vi "Operate LEDs.vi"(8 "error in (no error)":errorcluster, 10 "LED Panel":T1, 11 "COM port in":refnum<visa-resource-name>) -> (0 "error out":errorcluster, 3 "COM port out":refnum<visa-resource-name>)   [LabVIEW 2020]
uses:
  Controls/LED panel ---typedef.ctl
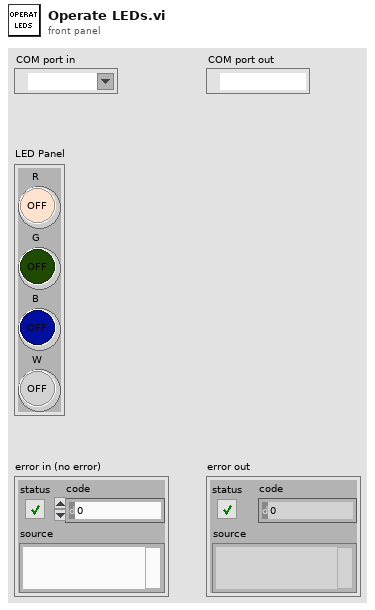
[diagram p1: front panel]
types:
  T1 = typedef "LED panel ---typedef.ctl" = cluster{"R":bool, "G":bool, "B":bool, "W":bool}
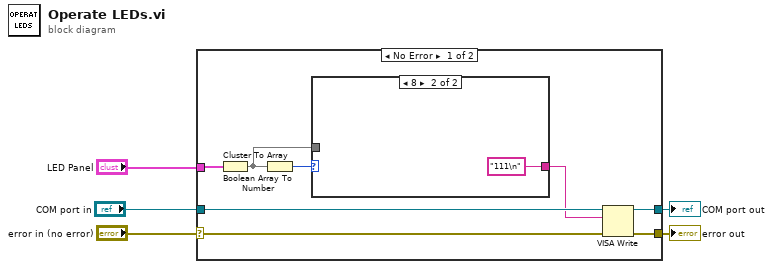
[diagram p0: block diagram]
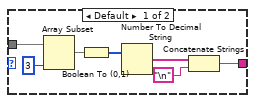
[diagram p2: hidden frame]
diagram:
  n1 = case shown="No Error" "error in (no error)" {
    selector: "error in (no error)" -> [w12 w23]
    tunnel: [w10 w23] -> w4
    tunnel: "LED Panel" -> [w13 _]
    tunnel: "COM port in" -> [w9 w22]
    tunnel: [w8 w22] -> w1
    frame No Error {
      n2 = Cluster To Array(cluster=w13) -> (array=w6:bool[])
      n3 = Boolean Array To Number(Boolean array=w6) -> (number=w11:u32)
      n4 = case shown="8" w11 {
        tunnel: [w14 "111\n"] -> w7
        tunnel: w6 -> [w20 _]
        frame Default {
          n5 = Array Subset(array=w20, length=3) -> (w18:bool[])  [unwired: 1 in]
          n6 = Boolean To (0,1)(Boolean=w18) -> (0, 1=w17:i16[])
          n7 = Number To Decimal String(number=w17) -> (decimal integer string=w16:string[])  [unwired: 1 in]
          n8 = Concatenate Strings(w16, "\n") -> (w14:string)
        }
        frame 8 {
        }
      }
      n9 = VISA Write(VISA resource name=w9, write buffer=w7, error in (no error)=w12) -> (VISA resource name out=w8:refnum<visa-resource-name>, error out=w10:errorcluster)  [unwired: 1 out]
    }
    frame Error {
    }
  }
  "error out" <- w4
  "COM port out" <- w1
